vi "Configure Output Power.vi"(0 "VISA resource name":refnum<visa-resource-name>, 5 "Platform Slot Number (10)":i16=10 min=-1 max=255, 7 "Output Power (0:MINimum)":i32(ring) items=["MINimum", "MAXimum", "DEFault", "User Defined Value"], 9 "User Defined Output Power Value (-15.000)":dbl=-15.0 format="%_5f", 11 "error in (no error)":errorcluster) -> (4 "VISA resource name out":refnum<visa-resource-name>, 15 "error out":errorcluster)   [LabVIEW 2018, in "LTB-1.lvlib" / "3150.lvlib"]
doc: "Configures the absolute output power to a specific value, in dBM."
uses:
  3150.lvlib
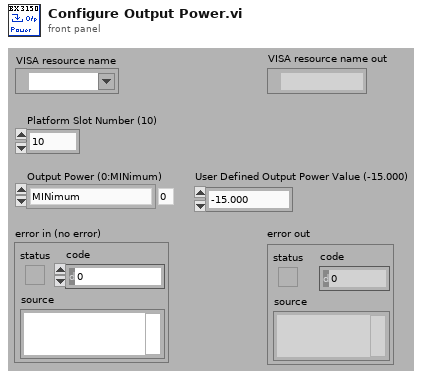
[diagram p1: front panel]
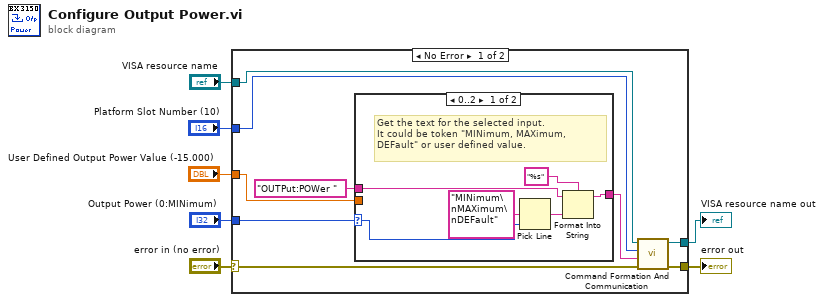
[diagram p0: block diagram]
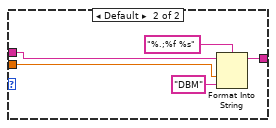
[diagram p2: hidden frame]
diagram:
  n1 = case shown="No Error" "error in (no error)" {
    selector: "error in (no error)" -> [w14 w29]
    tunnel: "VISA resource name" -> [w12 w28]
    tunnel: [w10 w29] -> w5
    tunnel: "Output Power (0:MINimum)" -> [w9 _]
    tunnel: "Platform Slot Number (10)" -> [w13 _]
    tunnel: [w11 w28] -> w2
    tunnel: "User Defined Output Power Value (-15.000)" -> [w8 _]
    frame No Error {
      n2 = case shown="0..2" w9 {
        selector: w9 -> [w18 _]
        tunnel: "OUTPut:POWer " ("Command") -> [w19 w26]
        tunnel: [w17 w25] -> w15
        tunnel: w8 -> [_ w23]
        frame 0..2 {
          # "Get the text for the selected input.\nIt could be token \"MINimum, MAXimum,\nDEFault\" or user defined value."
          n3 = Pick Line(multi-line string="MINimum\nMAXimum\nDEFault", line index=w18) -> (output string=w20:string)  [unwired: 1 out]
          n4 = Format Into String(format string="%s", initial string=w19, w20) -> (resulting string=w17:string)  [unwired: 1 in, 1 out]
        }
        frame Default {
          n5 = Format Into String(format string="%.;%f %s", initial string=w26, w23, "DBM") -> (resulting string=w25:string)  [unwired: 1 in, 1 out]
        }
      }
      n6 = call "Command Formation And Communication.vi"("error in (no error)"=w14, "Command"=w15, "Platform Slot Number"=w13, "VISA resource name"=w12) -> ("error out"=w10:errorcluster, "VISA resource name out"=w11:refnum<visa-resource-name>)  [unwired: 6 out]
    }
    frame Error {
    }
  }
  "VISA resource name out" <- w2
  "error out" <- w5
